vi "Get Ref.vi"(8 "error in":errorcluster, 11 "Session Handle In":T1) -> (0 "error out":errorcluster, 2 "Ref":T2, 3 "Session Handle Out":T1)   [LabVIEW 2018, in "Config Data.lvclass"]
uses:
  Config Data.lvclass
  <vilib>/MSR Consulting, LLC/General Reuse/Session APIs/_Session Fwk/Typedefs/Session Handle.ctl
  <vilib>/MSR Consulting, LLC/General Reuse/Session APIs/_Session Fwk/Session - Root.lvclass
  <vilib>/Utility/config.llb/Config Data RefNum.ctl
  C:/Program Files (x86)/National Instruments/LabVIEW 2018/vi.lib/MSR Consulting, LLC/General Reuse/Session APIs/_Session Fwk/Session - Root.lvclass
  Config Data.lvclass/Config Data.ctl
  Read Ref.vi
  <vilib>/Utility/config.llb/NI_LVConfig.lvlib
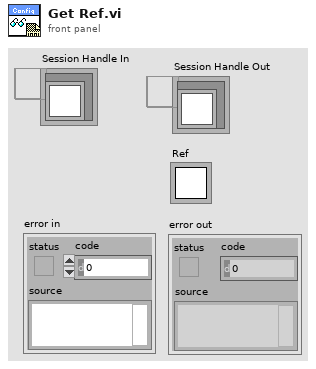
[diagram p1: front panel]
types:
  T1 = typedef "Session - Root.lvclass/Session Handle.ctl" = refnum<data-value>
  T2 = typedef "NI_LVConfig.lvlib/Config Data RefNum.ctl" = refnum<k1>
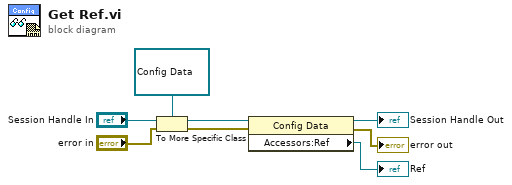
[diagram p0: block diagram]
diagram:
  n1 = To More Specific Class(target class=refnum<data-value> refnum ("Session Handle"), reference="Session Handle In", error in="error in") -> (specific class reference=w6:refnum<data-value>, error out=w4:errorcluster)
  n2 = property class="Config Data"(reference=w6, error in=w4) -> (reference out=→"Session Handle Out":refnum<data-value>, error out=→"error out":errorcluster, "Accessors:Ref"=→"Ref":T2)
